vi "Load.vi"(8 "error in":errorcluster, 10 "Source":string, 11 "PCAN-USB Read-Write Raw CAN Frame Strategy in":refnum<class "PCAN Base Strategy.lvclass">) -> (0 "error out":errorcluster, 3 "PCAN-USB Read-Write Raw CAN Frame Strategy out":refnum<class "PCAN Base Strategy.lvclass">)   [LabVIEW 2024, in "PCAN Base Strategy.lvclass"]
uses:
  PCAN Base Strategy.lvclass
  PCAN Base Strategy.lvclass/PCAN Base Strategy.ctl
  Source/Config from JSON/Config from JSON.lvclass
  D:/git/HAL/Source/Config from JSON/Config from JSON.lvclass
  D:/git/HAL/Source/Interfaces/IConfiguration/IConfiguration.lvclass
  Source/Config from Excel Table/Config from Excel Table.lvclass
  D:/git/HAL/Source/Config from Excel Table/Config from Excel Table.lvclass
  D:/git/HAL/Source/Interfaces/IClose/IClose.lvclass
  Source/Interfaces/IConfiguration/IConfiguration.lvclass
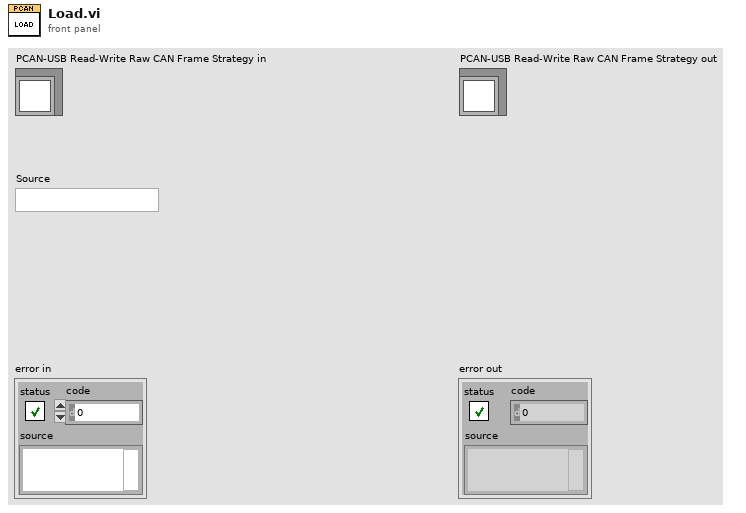
[diagram p1: front panel]
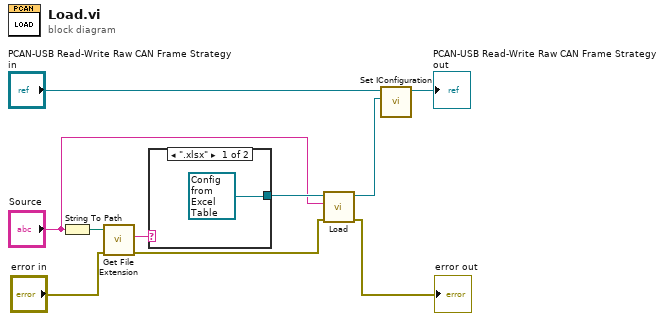
[diagram p0: block diagram]
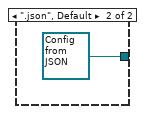
[diagram p2: hidden frame]
diagram:
  n1 = String To Path(string="Source") -> (path=w6:path)
  n2 = call <vilib>:"Get File Extension.vi"("error in (no error)"="error in", "file"=w6) -> ("error out"=w4:errorcluster, "lowercase file extension"=w3:string)  [unwired: 5 in, 3 out]
  n3 = case shown="\".xlsx\"" w3 {
    tunnel: [refnum<class "Config from Excel Table.lvclass"> refnum ("Config from Excel Table.lvclass") refnum<class "Config from JSON.lvclass"> refnum ("Config from JSON.lvclass")] -> w2
    frame ".xlsx" {
    }
    frame ".json", Default {
    }
  }
  n4 = call-dynamic "Load.vi"("error in"=w4, "Source"="Source", "IConfiguration in"=w2) -> ("error out"=→"error out":errorcluster, "IConfiguration out"=w7:refnum<class "IConfiguration.lvclass">)  [unwired: 7 in]
  n5 = call-dynamic "Set IConfiguration.vi"("IConfiguration"=w7, "PCAN-USB Read-Write Raw CAN Frame Strategy in"="PCAN-USB Read-Write Raw CAN Frame Strategy in") -> ("PCAN-USB Read-Write Raw CAN Frame Strategy out"=→"PCAN-USB Read-Write Raw CAN Frame Strategy out":refnum<class "PCAN Base Strategy.lvclass">)  [unwired: 9 in]
